vi "Utility_Calculate.vi"(4 "input_2":dbl, 6 "input_1":dbl, 7 "error in":errorcluster, 8 "units":enum16{"SI", "IP"}(ring), 9 "InpCode":T3(ring), 10 "Mixure Cluster":T1) -> (0 "error out":errorcluster, 3 "dataout":dbl[](array[numeric]))   [LabVIEW 2016]
doc: "Utility function that provides access to all of the functionality contained in the FLSH and SAT polymorphic VIs. \n\nPlease feel free to contact me if you have any questions .\nMy mail:ken_pop@tom.com yan.ding@jci.com"
uses:
  Ctl/Mixture Composition cluster_d.ctl
  Ctl/variable_refprop.ctl
  Ctl/FLSH_Inputs.ctl
  VIs/PSFLSHdll.vi
  VIs/HSFLSHdll.vi
  VIs/SATTdll.vi
  VIs/SATPdll.vi
  VIs/TPFLSHdll.vi
  VIs/THFLSHdll.vi
  VIs/TSFLSHdll.vi
  VIs/PHFLSHdll.vi
  VIs/PQFLSHdll.vi
  VIs/TQFLSHdll.vi
panel:
  out "INFO_OUT":T2
  out "n":i32
  out "wm":dbl
  out "x":dbl[](array[numeric])
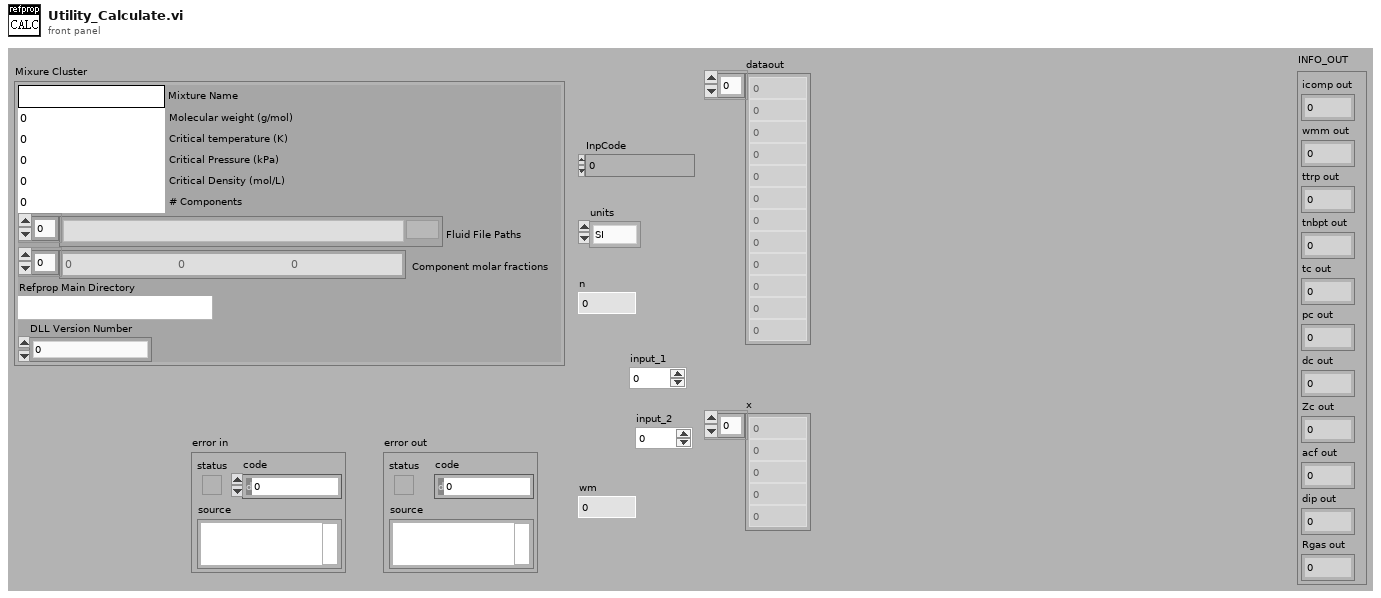
[diagram p1: front panel]
types:
  T1 = typedef "Mixture Composition cluster_d.ctl" = cluster{"Mixture Name":string, "Molecular weight (g/mol)":dbl, "Critical temperature (K)":dbl, "Critical Pressure (kPa)":dbl, "Critical Density (mol/L)":dbl, "# Components":i32, "Fluid File Paths":path[], "Component molar fractions":dbl[], "Refprop Main Directory":path, "DLL Version Number":dbl}
  T2 = cluster{"icomp out":i32, "wmm out":dbl, "ttrp out":dbl, "tnbpt out":dbl, "tc out":dbl, "pc out":dbl, "dc out":dbl, "Zc out":dbl, "acf out":dbl, "dip out":dbl, "Rgas out":dbl}
  T3 = enum16{"0", "PS", "HS", "T", "P", "TP", "TH", "TS", "PH", "PQ", "TQ"}
  T4 = typedef "FLSH_Inputs.ctl" = cluster{"t":dbl, "p":dbl, "e":dbl, "h":dbl, "s":dbl, "q":dbl, "z":dbl[], "kq":i32, "kr":i32, "D":dbl}
  T5 = typedef "variable_refprop.ctl" = cluster{"t":dbl, "p":dbl, "z":dbl[], "d":dbl, "D":dbl, "Dl":dbl, "Dv":dbl, "x":dbl[], "y":dbl[], "q":dbl, "e":dbl, "h":dbl, "s":dbl, "Cv":dbl, "Cp":dbl, "w":dbl, "ierr":i32, "herr":string, "i":i32, "z":dbl, "kq":i32, "kph":i32, "kr":i32, "nroot":i32, "k1":i32, "t1":dbl, "p1":dbl, "d1":dbl, "k2":i32, "t2":dbl, "p2":dbl, "d2":dbl, "k3":i32, "t3":dbl, "p3":dbl, "d3":dbl, "iGuess":dbl}
  T6 = typedef "FLSH_Outputs.ctl" = cluster{"t":dbl, "p":dbl, "D":dbl, "Dl":dbl, "Dv":dbl, "x":dbl[], "y":dbl[], "q":dbl, "e":dbl, "h":dbl, "s":dbl, "Cv":dbl, "Cp":dbl, "w":dbl, "ierr":i32, "herr":string, "herr_Length":i32}
  T7 = typedef "SAT_Outputs.ctl" = cluster{"D":dbl, "e":dbl, "h":dbl, "p":dbl, "s":dbl, "t":dbl, "q":dbl, "Dl":dbl, "Dv":dbl, "x":dbl[], "y":dbl[], "nroot":i32, "k1":i32, "t1":dbl, "p1":dbl, "d1":dbl, "k2":i32, "t2":dbl, "p2":dbl, "d2":dbl, "k3":i32, "t3":dbl, "p3":dbl, "d3":dbl, "ierr":i32, "herr":string, "herr_length":i32}
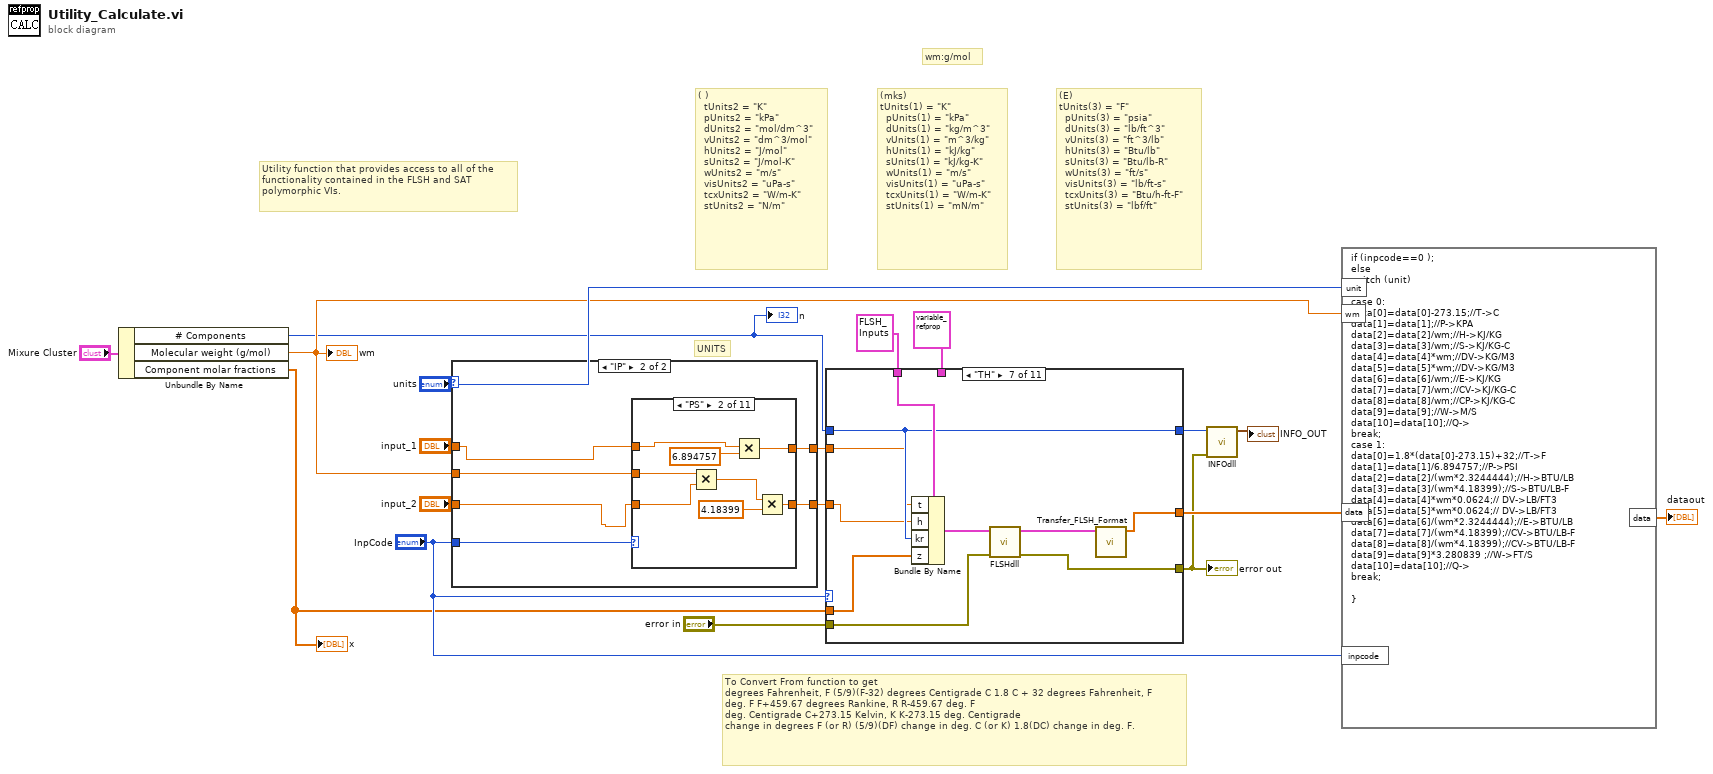
[diagram p0: block diagram]
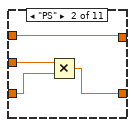
[diagram p4: hidden frame]
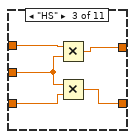
[diagram p5: hidden frame]
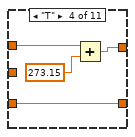
[diagram p6: hidden frame]
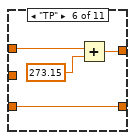
[diagram p7: hidden frame]
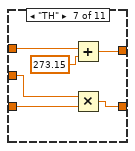
[diagram p8: hidden frame]
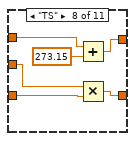
[diagram p9: hidden frame]
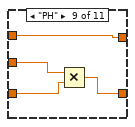
[diagram p10: hidden frame]
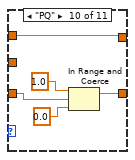
[diagram p11: hidden frame]
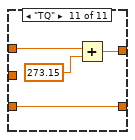
[diagram p12: hidden frame]
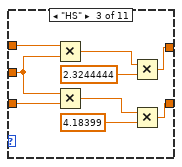
[diagram p14: hidden frame]
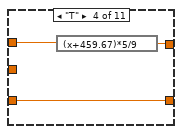
[diagram p15: hidden frame]
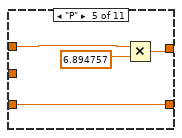
[diagram p16: hidden frame]
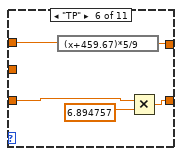
[diagram p17: hidden frame]
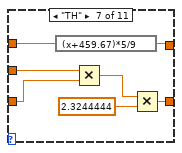
[diagram p18: hidden frame]
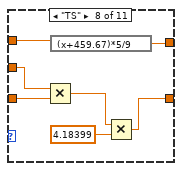
[diagram p19: hidden frame]
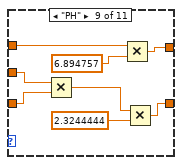
[diagram p20: hidden frame]
diagram:
  # "Utility function that provides access to all of the functionality contained in the FLSH and SAT polymorphic VIs."
  # "To Convert From function to get \ndegrees Fahrenheit, F (5/9)(F-32) degrees Centigrade C 1.8 C + 32 degrees Fahrenheit, F \ndeg. F F+459.67 degrees Rankine, R R-459.67 deg. F \ndeg. Centigrade C+273.15 Kelvin, K K-273.15 deg. Centigrade \nchange in degrees F (or R) (5/9)(DF) change in deg. C (or K) 1.8(DC) change in deg. F."
  # "(E)\ntUnits(3) = \"F\"\n  pUnits(3) = \"psia\"\n  dUnits(3) = \"lb/ft^3\"\n  vUnits(3) = \"ft^3/lb\"\n  hUnits(3) = \"Btu/lb\"\n  sUnits(3) = \"Btu/lb-R\"\n  wUnits(3) = \"ft/s\"\n  visUnits(3) = \"lb/ft-s\"\n  tcxUnits(3) = \"Btu/h-ft-F\"\n  stUnits(3) = \"lbf/ft\""
  # "(mks)\ntUnits(1) = \"K\"\n  pUnits(1) = \"kPa\"\n  dUnits(1) = \"kg/m^3\"\n  vUnits(1) = \"m^3/kg\"\n  hUnits(1) = \"kJ/kg\"\n  sUnits(1) = \"kJ/kg-K\"\n  wUnits(1) = \"m/s\"\n  visUnits(1) = \"uPa-s\"\n  tcxUnits(1) = \"W/m-K\"\n  stUnits(1) = \"mN/m\""
  # "( )\n  tUnits2 = \"K\"\n  pUnits2 = \"kPa\"\n  dUnits2 = \"mol/dm^3\"\n  vUnits2 = \"dm^3/mol\"\n  hUnits2 = \"J/mol\"\n  sUnits2 = \"J/mol-K\"\n  wUnits2 = \"m/s\"\n  visUnits2 = \"uPa-s\"\n  tcxUnits2 = \"W/m-K\"\n  stUnits2 = \"N/m\""
  # "wm:g/mol"
  # "UNITS"
  n1 = Unbundle By Name("Mixure Cluster") -> ("# Components"=w3:i32, "Molecular weight (g/mol)"=w7:dbl, "Component molar fractions"=w6:dbl[])
  "x" <- w6
  "wm" <- w7
  "n" <- w3
  n2 = case shown="\"IP\"" "units" {
    tunnel: "InpCode" -> [w24 w73]
    tunnel: "input_1" -> [w20 w72]
    tunnel: [w21 w76] -> w1
    tunnel: "input_2" -> [w19 w71]
    tunnel: [w23 w75] -> w15
    tunnel: w7 -> [w22 w74]
    frame "SI", Default {
      n3 = case shown="\"P\"" w24 {
        tunnel: [w26 w28 w33 w38 w41 w44 w50 w56 w59 w63 w69] -> w21
        tunnel: [w25 w29 w34 w36 w40 w42 w48 w54 w60 w64 w67] -> w23
        tunnel: w22 -> [_ w30 w35 _ _ _ w49 w55 w61 _ _]
        tunnel: w20 -> [w26 w28 w32 w37 w41 w43 w46 w53 w59 w63 w68]
        tunnel: w19 -> [w25 w27 w31 w36 w40 w42 w47 w52 w58 w62 w67]
        frame "0", Default {
        }
        frame "PS" {
          n4 = Multiply(x=w30, y=w27) -> (x*y=w29:dbl)
        }
        frame "HS" {
          n5 = Multiply(x=w32, y=w35) -> (x*y=w33:dbl)
          n6 = Multiply(x=w35, y=w31) -> (x*y=w34:dbl)
        }
        frame "T" {
          n7 = Add(x=w37, y=273.15) -> (x+y=w38:dbl)
        }
        frame "P" {
        }
        frame "TP" {
          n8 = Add(x=w43, y=273.15) -> (x+y=w44:dbl)
        }
        frame "TH" {
          n9 = Add(x=w46, y=273.15) -> (x+y=w50:dbl)
          n10 = Multiply(x=w49, y=w47) -> (x*y=w48:dbl)
        }
        frame "TS" {
          n11 = Add(x=w53, y=273.15) -> (x+y=w56:dbl)
          n12 = Multiply(x=w55, y=w52) -> (x*y=w54:dbl)
        }
        frame "PH" {
          n13 = Multiply(x=w61, y=w58) -> (x*y=w60:dbl)
        }
        frame "PQ" {
          n14 = In Range and Coerce(upper limit=1.0 ("上限"), x=w62, lower limit=0.0 ("下限")) -> (coerced(x)=w64:dbl)  [unwired: 1 out]
        }
        frame "TQ" {
          n15 = Add(x=w68, y=273.15) -> (x+y=w69:dbl)
        }
      }
    }
    frame "IP" {
      n16 = case shown="\"PS\"" w73 {
        tunnel: w72 -> [w78 w80 w88 w97 w100 w104 w109 w115 w122 w130 w138]
        tunnel: [w78 w84 w89 w98 w101 w105 w110 w117 w127 w132 w139] -> w76
        tunnel: w71 -> [w77 w79 w87 w96 w99 w103 w108 w116 w123 w131 w137]
        tunnel: [w77 w81 w92 w96 w99 w106 w111 w118 w124 w134 w137] -> w75
        tunnel: w74 -> [_ w86 w95 _ _ _ w114 w121 w129 _ _]
        frame "0", Default {
        }
        frame "PS" {
          n17 = Multiply(x=w86, y=w79) -> (x*y=w82:dbl)
          n18 = Multiply(x=w80, y=6.894757) -> (x*y=w84:dbl)
          n19 = Multiply(x=w82, y=4.18399) -> (x*y=w81:dbl)
        }
        frame "HS" {
          n20 = Multiply(x=w88, y=w95) -> (x*y=w90:dbl)
          n21 = Multiply(x=w95, y=w87) -> (x*y=w93:dbl)
          n22 = Multiply(x=w90, y=2.3244444) -> (x*y=w89:dbl)
          n23 = Multiply(x=w93, y=4.18399) -> (x*y=w92:dbl)
        }
        frame "T" {
          n24 = expression code="(x+459.67)*5/9"(w97) -> (w98:dbl)
        }
        frame "P" {
          n25 = Multiply(x=w100, y=6.894757) -> (x*y=w101:dbl)
        }
        frame "TP" {
          n26 = expression code="(x+459.67)*5/9"(w104) -> (w105:dbl)
          n27 = Multiply(x=w103, y=6.894757) -> (x*y=w106:dbl)
        }
        frame "TH" {
          n28 = expression code="(x+459.67)*5/9"(w109) -> (w110:dbl)
          n29 = Multiply(x=w114, y=w108) -> (x*y=w112:dbl)
          n30 = Multiply(x=w112, y=2.3244444) -> (x*y=w111:dbl)
        }
        frame "TS" {
          n31 = Multiply(x=w121, y=w116) -> (x*y=w119:dbl)
          n32 = expression code="(x+459.67)*5/9"(w115) -> (w117:dbl)
          n33 = Multiply(x=w119, y=4.18399) -> (x*y=w118:dbl)
        }
        frame "PH" {
          n34 = Multiply(x=w129, y=w123) -> (x*y=w125:dbl)
          n35 = Multiply(x=w122, y=6.894757) -> (x*y=w127:dbl)
          n36 = Multiply(x=w125, y=2.3244444) -> (x*y=w124:dbl)
        }
        frame "PQ" {
          n37 = In Range and Coerce(upper limit=1.0 ("上限"), x=w131, lower limit=0.0 ("下限")) -> (coerced(x)=w134:dbl)  [unwired: 1 out]
          n38 = Multiply(x=w130, y=6.894757) -> (x*y=w132:dbl)
        }
        frame "TQ" {
          n39 = expression code="(x+459.67)*5/9"(w138) -> (w139:dbl)
        }
      }
    }
  }
  n40 = case shown="\"TH\"" "InpCode" {
    tunnel: w6 -> [_ w150 w161 w171 w179 w188 w199 w209 w220 w229 w239]
    tunnel: "error in" -> [w144 w154 w163 w173 w181 w192 w201 w212 w222 w231 w241]
    tunnel: [w144 w153 w162 w172 w182 w190 w200 w211 w221 w230 w240] -> w2
    tunnel: w1 -> [_ w145 w156 w165 w174 w184 w194 w204 w213 w224 w233]
    tunnel: w15 -> [_ w146 w155 _ _ w183 w193 w203 w214 w223 w234]
    tunnel: w3 -> [w140 w149 w160 w166 w175 w185 w197 w207 w217 w227 w237]
    tunnel: [w141 w148 w158 w167 w176 w187 w195 w206 w215 w225 w236] -> w14
    tunnel: T5 {"t"=0.0, "p"=0.0, "z"=[0.0, 0.0, 0.0, 0.0, 0.0, 0.0, 0.0, 0.0, 0.0, 0.0, 0.0, 0.0, 0.0, 0.0, 0.0, 0.0, 0.0, 0.0, 0.0, 0.0], "d"=0.0, "D"=0.0, "Dl"=0.0, "Dv"=0.0, "x"=[0.0, 0.0, 0.0, 0.0, 0.0, 0.0, 0.0, 0.0, 0.0, 0.0, 0.0, 0.0, 0.0, 0.0, 0.0, 0.0, 0.0, 0.0, 0.0, 0.0], "y"=[0.0, 0.0, 0.0, 0.0, 0.0, 0.0, 0.0, 0.0, 0.0, 0.0, 0.0, 0.0, 0.0, 0.0, 0.0, 0.0, 0.0, 0.0, 0.0, 0.0], "q"=0.0, "e"=0.0, "h"=0.0, "s"=0.0, "Cv"=0.0, "Cp"=0.0, "w"=0.0, "ierr"=0, "herr"="", "i"=0, "z"=0.0, "kq"=0, "kph"=0, "kr"=0, "nroot"=0, "k1"=0, "t1"=0.0, "p1"=0.0, "d1"=0.0, "k2"=0, "t2"=0.0, "p2"=0.0, "d2"=0.0, "k3"=0, "t3"=0.0, "p3"=0.0, "d3"=0.0, "iGuess"=0.0} ("variable") -> [_ _ _ _ _ _ _ _ _ _ _]
    tunnel: [w140 w149 w160 w166 w175 w185 w197 w207 w217 w227 w237] -> w4
    tunnel: T4 {"t"=0.0, "p"=0.0, "e"=0.0, "h"=0.0, "s"=0.0, "q"=0.0, "z"=[0.0, 0.0, 0.0, 0.0, 0.0, 0.0, 0.0, 0.0, 0.0, 0.0, 0.0, 0.0, 0.0, 0.0, 0.0, 0.0, 0.0, 0.0, 0.0, 0.0], "kq"=0, "kr"=0, "D"=0.0} ("FLSH Inputs") -> [_ w151 w157 _ _ w189 w198 w210 w219 w228 w238]
    frame "0", Default {
      n41 = Initialize Array(0.0 ("元素"), 10 ("维数大小")) -> (w141:dbl[])
    }
    frame "PS" {
      n42 = Bundle By Name(cluster=w151, "p"=w145, "s"=w146, "z"=w150) -> (w152:T4)
      n43 = call-poly "FLSHdll.vi"("error in (no error)"=w154, "FLSH Inputs"=w152) -> ("error out"=w153:errorcluster, "FLSH Outputs"=w147:T6)  [unwired: 8 in]
      n44 = call "Transfer_FLSH_Format.vi"("FLSH Outputs"=w147) -> ("Array out"=w148:dbl[])  [unwired: 10 in]
    }
    frame "HS" {
      n45 = Bundle By Name(cluster=w157, "h"=w156, "s"=w155, "z"=w161) -> (w164:T4)
      n46 = call-poly "FLSHdll.vi"("error in (no error)"=w163, "FLSH Inputs"=w164) -> ("error out"=w162:errorcluster, "FLSH Outputs"=w159:T6)  [unwired: 8 in]
      n47 = call "Transfer_FLSH_Format.vi"("FLSH Outputs"=w159) -> ("Array out"=w158:dbl[])  [unwired: 10 in]
    }
    frame "T" {
      n48 = Bundle By Name(cluster=cluster{"t":dbl, "z":dbl[], "kph":u16} {"t"=0.0, "z"=[0.0, 0.0, 0.0, 0.0, 0.0, 0.0, 0.0, 0.0, 0.0, 0.0, 0.0, 0.0, 0.0, 0.0, 0.0, 0.0, 0.0, 0.0, 0.0, 0.0], "kph"=2} ("SAT Inputs"), "t"=w165, "z"=w171, "kph"=w166) -> (w170:cluster{"t":dbl, "z":dbl[], "kph":u16})
      n49 = call-poly "SAT.vi"("error in (no error)"=w173, "SAT Inputs"=w170) -> ("error out"=w172:errorcluster, "SAT Outputs"=w168:T7)  [unwired: 8 in]
      n50 = call "Transfer_SAT_Format.vi"("SAT Outputs"=w168) -> ("Array out"=w167:dbl[])  [unwired: 10 in]
    }
    frame "P" {
      n51 = Bundle By Name(cluster=cluster{"p":dbl, "z":dbl[], "kph":u16} {"p"=0.0, "z"=[0.0, 0.0, 0.0, 0.0, 0.0, 0.0, 0.0, 0.0, 0.0, 0.0, 0.0, 0.0, 0.0, 0.0, 0.0, 0.0, 0.0, 0.0, 0.0, 0.0], "kph"=4} ("SAT Inputs"), "p"=w174, "z"=w179, "kph"=w175) -> (w178:cluster{"p":dbl, "z":dbl[], "kph":u16})
      n52 = call-poly "SAT.vi"("error in (no error)"=w181, "SAT Inputs"=w178) -> ("error out"=w182:errorcluster, "SAT Outputs"=w177:T7)  [unwired: 8 in]
      n53 = call "Transfer_SAT_Format.vi"("SAT Outputs"=w177) -> ("Array out"=w176:dbl[])  [unwired: 10 in]
    }
    frame "TP" {
      n54 = Bundle By Name(cluster=w189, "t"=w184, "p"=w183, "z"=w188) -> (w191:T4)
      n55 = call-poly "FLSHdll.vi"("error in (no error)"=w192, "FLSH Inputs"=w191) -> ("error out"=w190:errorcluster, "FLSH Outputs"=w186:T6)  [unwired: 8 in]
      n56 = call "Transfer_FLSH_Format.vi"("FLSH Outputs"=w186) -> ("Array out"=w187:dbl[])  [unwired: 10 in]
    }
    frame "TH" {
      n57 = Bundle By Name(cluster=w198, "t"=w194, "h"=w193, "kr"=w197, "z"=w199) -> (w202:T4)
      n58 = call-poly "FLSHdll.vi"("error in (no error)"=w201, "FLSH Inputs"=w202) -> ("error out"=w200:errorcluster, "FLSH Outputs"=w196:T6)  [unwired: 8 in]
      n59 = call "Transfer_FLSH_Format.vi"("FLSH Outputs"=w196) -> ("Array out"=w195:dbl[])  [unwired: 10 in]
    }
    frame "TS" {
      n60 = Bundle By Name(cluster=w210, "t"=w204, "s"=w203, "kr"=w207, "z"=w209) -> (w208:T4)
      n61 = call-poly "FLSHdll.vi"("error in (no error)"=w212, "FLSH Inputs"=w208) -> ("error out"=w211:errorcluster, "FLSH Outputs"=w205:T6)  [unwired: 8 in]
      n62 = call "Transfer_FLSH_Format.vi"("FLSH Outputs"=w205) -> ("Array out"=w206:dbl[])  [unwired: 10 in]
    }
    frame "PH" {
      n63 = Bundle By Name(cluster=w219, "p"=w213, "h"=w214, "z"=w220) -> (w218:T4)
      n64 = call-poly "FLSHdll.vi"("error in (no error)"=w222, "FLSH Inputs"=w218) -> ("error out"=w221:errorcluster, "FLSH Outputs"=w216:T6)  [unwired: 8 in]
      n65 = call "Transfer_FLSH_Format.vi"("FLSH Outputs"=w216) -> ("Array out"=w215:dbl[])  [unwired: 10 in]
    }
    frame "PQ" {
      n66 = Bundle By Name(cluster=w228, "p"=w224, "q"=w223, "kq"=w227, "z"=w229) -> (w232:T4)
      n67 = call-poly "FLSHdll.vi"("error in (no error)"=w231, "FLSH Inputs"=w232) -> ("error out"=w230:errorcluster, "FLSH Outputs"=w226:T6)  [unwired: 8 in]
      n68 = call "Transfer_FLSH_Format.vi"("FLSH Outputs"=w226) -> ("Array out"=w225:dbl[])  [unwired: 10 in]
    }
    frame "TQ" {
      n69 = Bundle By Name(cluster=w238, "t"=w233, "q"=w234, "kq"=w237, "z"=w239) -> (w242:T4)
      n70 = call-poly "FLSHdll.vi"("error in (no error)"=w241, "FLSH Inputs"=w242) -> ("error out"=w240:errorcluster, "FLSH Outputs"=w235:T6)  [unwired: 8 in]
      n71 = call "Transfer_FLSH_Format.vi"("FLSH Outputs"=w235) -> ("Array out"=w236:dbl[])  [unwired: 10 in]
    }
  }
  "error out" <- w2
  n72 = call "INFOdll.vi"("error in (no error)"=w2, "icomp"=w4) -> ("INFO_OUT"=→"INFO_OUT":T2)  [unwired: 8 in, 1 out]
  n73 = formula code="if (inpcode==0 );\nelse\nswitch (unit)\n{\ncase 0:\ndata[0]=data[0]-273.15;//T->C\ndata[1]=data[1];//P->KPA\ndata[2]=data[2]/wm;//H->KJ/KG\ndata[3]=data[3]/wm;//S->KJ/KG-C\ndata[4]=data[4]*wm;//DV->KG/M3\ndata[5]=data[5]*wm;//DV->KG/M3\ndata[6]=data[6]/wm;//E->KJ/KG\ndata[7]=data[7]/wm;//CV->KJ/KG-C\ndata[8]=data[8]/wm;//CP->KJ/KG-C\ndata[9]=data[9];//W->M/S\ndata[10]=data[10];//Q->\nbreak;\ncase 1:\ndata[0]=1.8*(data[0]-273.15)+32;//T->F\ndata[1]=data[1]/6.894757;//P->PSI\ndata[2]=data[2]/(wm*2.3244444);//H->BTU/LB\ndata[3]=data[3]/(wm*4.18399);//S->BTU/LB-F\ndata[4]=data[4]*wm*0.0624;// DV->LB/FT3\ndata[5]=data[5]*wm*0.0624;// DV->LB/FT3\ndata[6]=data[6]/(wm*2.3244444);//E->BTU/LB\ndata[7]=data[7]/(wm*4.18399);//CV->BTU/LB-F\ndata[8]=data[8]/(wm*4.18399);//CV->BTU/LB-F\ndata[9]=data[9]*3.280839 ;//W->FT/S\ndata[10]=data[10];//Q->\nbreak;\n\n}"("data"=w14, "unit"="units", "inpcode"="InpCode", "wm"=w7) -> ("data"=→"dataout":dbl[])
